vi "Get Excel Value.vi"(6 "SheetName(\"\")":string, 8 "error in (no error)":errorcluster, 9 "End":cluster{"Column":i32, "Row":i32}={"Column"=8, "Row"=7}, 10 "Start":cluster{"Column":i32, "Row":i32}={"Column"=1, "Row"=1}, 11 "path":path) -> (0 "error out":errorcluster, 2 "Excel_Value":variant)   [LabVIEW 2015]
uses:
  Private Methods/OpenXL_WorkSheet By Name.vi
  Private Methods/GetXL_CellValues_2D_String.vi
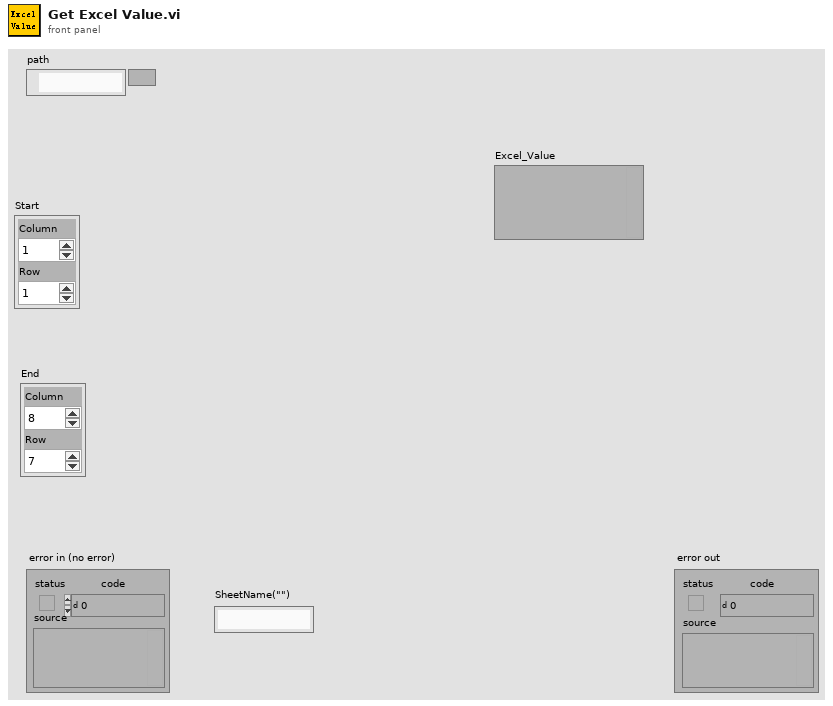
[diagram p1: front panel]
types:
  T1 = cluster{"Excel._Application":refnum<k7>, "Workbooks":refnum<k7>}
  T2 = cluster{"Excel._Application":refnum<k7>, "Workbooks":refnum<k7>, "Open":refnum<k7>}
  T3 = cluster{"Excel._Application":refnum<k7>, "Workbooks":refnum<k7>, "Open":refnum<k7>, "Worksheets":refnum<k7>, "Excel._Worksheet":refnum<k7>}
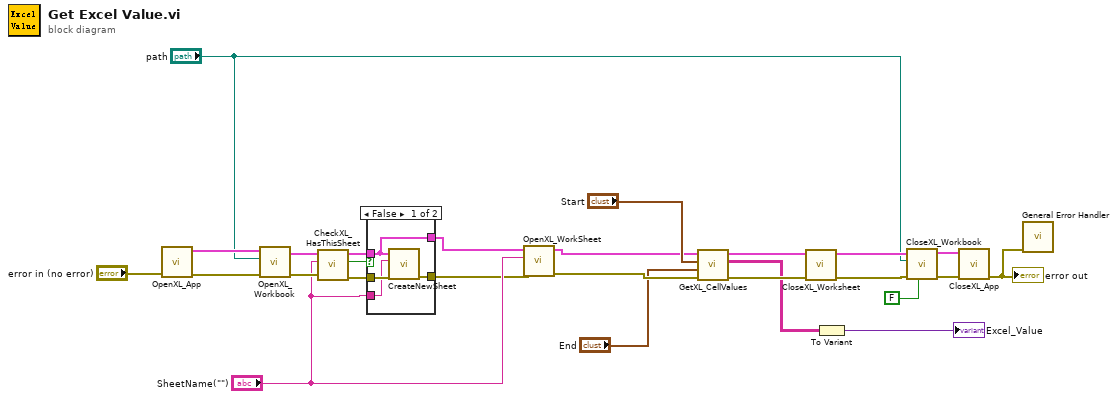
[diagram p0: block diagram]
diagram:
  n1 = call "OpenXL_App.vi"("error in (no error)"="error in (no error)") -> ("error out"=w25:errorcluster, "Refnum Cluster"=w26:T1)  [unwired: 9 in]
  n2 = call "OpenXL_Workbook.vi"("error in"=w25, "path"="path", "Refnum Cluster In"=w26) -> ("error out"=w7:errorcluster, "Refnum Cluster Out"=w8:T2)  [unwired: 7 in]
  n3 = call "CheckXL_HasThisSheet.vi"("error in (no error)"=w7, "SheetName(\"\")"="SheetName(\"\")", "Refnum Cluster In"=w8) -> ("error out"=w4:errorcluster, "Find(False)"=w6:bool, "Refnum Out"=w5:T2)  [unwired: 6 in]
  n4 = case shown="False" w6 {
    tunnel: w5 -> [w27 w32]
    tunnel: w4 -> [w30 w31]
    tunnel: "SheetName(\"\")" -> [w29 _]
    tunnel: [w28 w31] -> w1
    tunnel: [w27 w32] -> w2
    frame False {
      n5 = call "CreateNewSheet.vi"("error in (no error)"=w30, "SheetName"=w29, "Refnum Cluster In"=w27) -> ("error out"=w28:errorcluster)  [unwired: 7 in, 1 out]
    }
    frame True {
    }
  }
  n6 = call-poly "OpenXL_WorkSheet.vi"("error in (no error)"=w1, "SheetName(\"\")"="SheetName(\"\")", "Refnum Cluster In"=w2) -> ("error out"=w16:errorcluster, "Refnum Cluster Out"=w14:T3)  [unwired: 7 in]
  n7 = call-poly "GetXL_CellValues.vi"("error in"=w16, "End"="End", "Start"="Start", "Refnum Cluster In"=w14) -> ("error out"=w24:errorcluster, "data"=w13:string[][], "Refnum Cluster Out"=w23:T3)  [unwired: 5 in]
  n8 = call "CloseXL_Worksheet.vi"("error in (no error)"=w24, "Refnum Cluster In"=w23) -> ("error out"=w21:errorcluster, "Refnum Cluster Out"=w22:T2)  [unwired: 8 in]
  n9 = To Variant(anything=w13) -> (Variant=→"Excel_Value":variant)
  n10 = call "CloseXL_Workbook.vi"("Save? (F)"=FALSE, "error in (no error)"=w21, "path"="path", "Refnum Cluster In"=w22) -> ("error out"=w19:errorcluster, "Refnum Cluster Out"=w20:T1)  [unwired: 6 in]
  n11 = call "CloseXL_App.vi"("error in (no error)"=w19, "Refnum Cluster In"=w20) -> ("error out"=w9:errorcluster)  [unwired: 9 in]
  "error out" <- w9
  n12 = call <vilib>:"General Error Handler.vi"("error in (no error)"=w9) -> ()  [unwired: 10 in, 5 out]
